vi "Clear Pointer Data.vi"(8 "error in (no error)":errorcluster, 9 "offset (0)":u64 format="%d bytes", 10 "length (-1: rest)":i64=-1 format="%d bytes", 11 "Pointer in":refnum<class "Pointer.lvclass">) -> (0 "error out":errorcluster, 3 "Pointer out":refnum<class "Pointer.lvclass">)   [LabVIEW 2017, in "Memory Manager.lvlib" / "Pointer.lvclass"]
doc: "Sets the subset of bytes specified by <b>offset</b> and <b>length</b> within the provided <b>pointer</b> to zero.\n\n<b>Note:</b> This VI is <b>safe</b>, meaning it performs null pointer and bounds checks to prevent invaid memory access."
uses:
  Pointer.lvclass
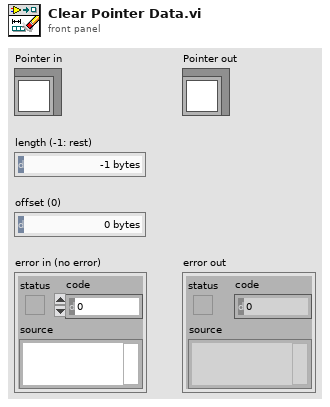
[diagram p1: front panel]
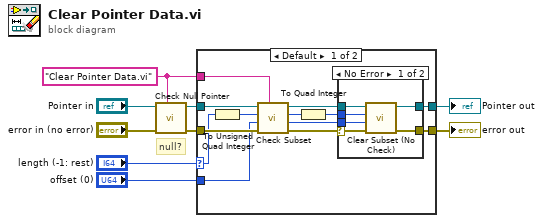
[diagram p0: block diagram]
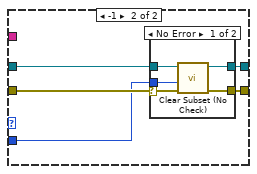
[diagram p3: hidden frame]
diagram:
  w5 = "Clear Pointer Data.vi" ("source vi name")
  # "null?"
  n1 = call "Check Null Pointer.vi"("source vi name"=w5, "error in (no error)"="error in (no error)", "Pointer in"="Pointer in") -> ("error out"=w9:errorcluster, "Pointer out"=w2:refnum<class "Pointer.lvclass">)  [unwired: 7 in]
  n2 = case shown="Default" "length (-1: rest)" {
    selector: "length (-1: rest)" -> [w21 _]
    tunnel: w9 -> [w22 w35]
    tunnel: w5 -> [w20 _]
    tunnel: [w16 w34] -> w4
    tunnel: [w15 w33] -> w3
    tunnel: w2 -> [w13 w32]
    tunnel: "offset (0)" -> [w10 w31]
    frame Default {
      n3 = To Unsigned Quad Integer(1:w21) -> (0:w12:u64)
      n4 = call "Check Subset.vi"("source vi name"=w20, "error in (no error)"=w22, "offset (0)"=w10, "length"=w12, "Pointer in"=w13) -> ("error out"=w14:errorcluster, "offset out"=w17:u64, "length"=w18:u64, "Pointer out"=w19:refnum<class "Pointer.lvclass">)  [unwired: 3 in]
      n5 = To Quad Integer(1:w18) -> (0:w11:i64)
      n6 = case shown="No Error" w14 {
        selector: w14 -> [w23 w29]
        tunnel: w19 -> [w28 w30]
        tunnel: w11 -> [w27 _]
        tunnel: w17 -> [w26 _]
        tunnel: [w25 w30] -> w16
        tunnel: [w24 w29] -> w15
        frame No Error {
          n7 = call "Clear Subset (No Check).vi"("error in (no error)"=w23, "offset (0)"=w26, "length (-1: rest)"=w27, "Pointer in"=w28) -> ("error out"=w24:errorcluster, "Pointer out"=w25:refnum<class "Pointer.lvclass">)  [unwired: 6 in]
        }
        frame Error {
        }
      }
    }
    frame -1 {
      n8 = case shown="No Error" w35 {
        selector: w35 -> [w36 w41]
        tunnel: w32 -> [w40 w42]
        tunnel: w31 -> [w39 _]
        tunnel: [w38 w42] -> w34
        tunnel: [w37 w41] -> w33
        frame No Error {
          n9 = call "Clear Subset (No Check).vi"("error in (no error)"=w36, "offset (0)"=w39, "Pointer in"=w40) -> ("error out"=w37:errorcluster, "Pointer out"=w38:refnum<class "Pointer.lvclass">)  [unwired: 7 in]
        }
        frame Error {
        }
      }
    }
  }
  "error out" <- w3
  "Pointer out" <- w4
